vi "Begin.vi"(8 "error in":errorcluster) -> (0 "error out":errorcluster)   [LabVIEW 2015]
doc: "Called before other user functions, this VI is expected to open initial I/O refnums, load in file data, and do all program initialization. Notice that the <B>error out</B> terminal is simply used for data flow. Wiring it to other structures or subVIs ensures that this VI runs first."
uses:
  <vilib>/Rock Robotics/WPI/DriverStation/WPI_DriverStationRobotMode2.ctl
  <vilib>/Rock Robotics/WPI/Joystick/WPI_JoystickDeviceEnum.ctl
  <vilib>/Rock Robotics/WPI/Solenoid/WPI_SolenoidChannel.ctl
  <vilib>/Rock Robotics/WPI/CAN/TalonSRX/WPI_CANTalonSRX_APIControlMode.ctl
  <vilib>/Rock Robotics/WPI/CAN/TalonSRX/WPI_CANTalonSRX_BrakeOverride.ctl
  <vilib>/Rock Robotics/SystemInterfaces/AI/FPGA_AIChannel.ctl
  <vilib>/Rock Robotics/SystemInterfaces/DIO/FPGA_DIOChannel.ctl
  <vilib>/Rock Robotics/SystemInterfaces/DIO/FPGA_DIOPWMChannel.ctl
  <vilib>/Rock Robotics/WPI/CAN/TalonSRX/WPI_CANTalonSRX_APIFeedbackSelect.ctl
  <vilib>/Rock Robotics/SystemInterfaces/spilib/spi_bus.ctl
  navX-MXP Library/COMMON/TypeDefs/Value TypeDefs/navX Interface Protocol.ctl
  navX-MXP Library/COMMON/TypeDefs/Value TypeDefs/navX Update Rate.ctl
  Robot Global Data.vi
  <vilib>/Rock Robotics/WPI/Utilities/WPI_GetSetVariantRefNum.vi
  <vilib>/Rock Robotics/WPI/Solenoid/WPI_SolenoidOpenSingle.vi
  <vilib>/Rock Robotics/WPI/MotorControl/WPI_MotorControlOpenCANTalonSRX.vi
  <vilib>/Rock Robotics/WPI/Ultrasonic/WPI_SonarSRF04DigitalOpen.vi
  <vilib>/Rock Robotics/WPI/Ultrasonic/WPI_SonarSRF04DigitalRefNum Registry Set.vi
  <vilib>/Rock Robotics/WPI/MotorControl/WPI_MotorControlOpen VictorSP.vi
  <vilib>/Rock Robotics/WPI/Counter/WPI_CounterDigitalInputToDigitalSource.vi
  <vilib>/Rock Robotics/WPI/Camera/WPI_CameraWhite Balance Values.ctl
  <vilib>/Rock Robotics/WPI/Camera/WPI_CameraExposure Values.ctl
  navX-MXP Library/navX-MXP IMU.lvlib
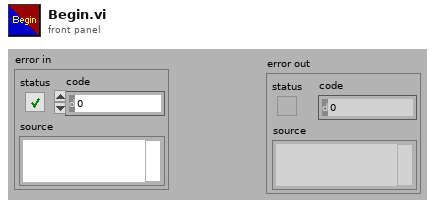
[diagram p1: front panel]
types:
  T1 = typedef "WPI_CANTalonSRX_APIFeedbackSelect.ctl" = enum16{"Digital Quadrature Encoder", "Analog Potentiometer", "Analog Encoder", "Count on Quad-A (Rising-Edge)", "Count on Quad-A (Falling-Edge)", "CTR Magnetic Enc (Absolute)", "CTR Magnetic Enc (Relative)", "Pulse Width"}
  T2 = typedef "FPGA_DIOPWMChannel.ctl" = enum8{"PWM 0", "PWM 1", "PWM 2", "PWM 3", "PWM 4", "PWM 5", "PWM 6", "PWM 7", "PWM 8", "PWM 9", "PWM MXP 0", "PWM MXP 1", "PWM MXP 2", "PWM MXP 3", "PWM MXP 4", "PWM MXP 5", "PWM MXP 6", "PWM MXP 7", "PWM MXP 8", "PWM MXP 9", "Invalid"}
  T3 = typedef "FPGA_DIOChannel.ctl" = enum8{"DIO 0", "DIO 1", "DIO 2", "DIO 3", "DIO 4", "DIO 5", "DIO 6", "DIO 7", "DIO 8", "DIO 9", "DIO MXP 0", "DIO MXP 1", "DIO MXP 2", "DIO MXP 3", "DIO MXP 4", "DIO MXP 5", "DIO MXP 6", "DIO MXP 7", "DIO MXP 8", "DIO MXP 9", "DIO MXP 10", "DIO MXP 11", "DIO MXP 12", "DIO MXP 13", "DIO MXP 14", "DIO MXP 15", "Invalid"}
  T4 = typedef "WPI_CANTalonSRX_BrakeOverride.ctl" = enum8{"No Override", "Override to Coast", "Override to Brake"}
  T5 = typedef "WPI_SolenoidChannel.ctl" = enum8{"Solenoid 0", "Solenoid 1", "Solenoid 2", "Solenoid 3", "Solenoid 4", "Solenoid 5", "Solenoid 6", "Solenoid 7", "Invalid"}
  T6 = typedef "WPI_CANTalonSRX_APIControlMode.ctl" = enum8{"Percent VBus", "Speed", "Position", "Slave", "Unchanged / Invalid", "Voltage Compensation", "Current", "Motion Profile"}
  T7 = typedef "FPGA_AIChannel.ctl" = enum8{"AI 0", "AI 1", "AI 2", "AI 3", "AI MXP 0", "AI MXP 1", "AI MXP 2", "AI MXP 3", "Invalid"}
  T8 = typedef "WPI_JoystickDeviceEnum.ctl" = enum16{"USB 0", "USB 1", "USB 2", "USB 3", "USB 4", "USB 5"}
  T9 = typedef "WPI_DriverStationRobotMode2.ctl" = enum16{"Autonomous Disabled", "Autonomous Enabled", "Teleop Disabled", "Teleop Enabled", "Disconnected", "Finish", "Test Disabled", "Test Enabled", "Emergency Stopped"}
  T10 = typedef "navX-MXP IMU.lvlib/navX Update Rate.ctl" = u8
  T11 = typedef "navX-MXP IMU.lvlib/navX Interface Protocol.ctl" = enum16{"SPI", "I2C"}
  T12 = typedef "spi_bus.ctl" = enum16{"SPI On-Board, CS0", "SPI On-Board, CS1", "SPI On-Board, CS2", "SPI On-Board, CS3", "SPI MXP", "Invalid"}
  T13 = typedef "navX-MXP IMU.lvlib/navX Device TypeDef.ctl" = cluster{"navX Interface Protocol":T11, "navX Interface Protocol TypeDefs":cluster{"SPIDevRef":T14, "I2CDevRef":T15}, "navX System Information":cluster{"Board Information":T17, "Status":T18, "Offsets":T22}, "navX Common Information":cluster{"Update Rate (4Hz-60Hz)":T10, "refnum name":string, "error":errorcluster}}
  T14 = typedef "WPI_SPIDevRef.ctl" = cluster{"DevStatus":errorcluster, "Handle":i32, "SPI Bus":T12}
  T15 = typedef "WPI_I2CDevRef.ctl" = cluster{"DevStatus":errorcluster, "Device Address":u8, "Handle":i32, "I2C Bus":T16}
  T16 = typedef "i2c_bus.ctl" = enum16{"I2C On-Board", "I2C MXP", "Invalid"}
  T17 = typedef "navX-MXP IMU.lvlib/navX Board Information.ctl" = cluster{"WhoAmI (50 | 0x32)":u8, "Board Revision":u8, "Firmware Major Version":u8, "Firmware Minor Version":u8}
  T18 = typedef "navX-MXP IMU.lvlib/navX Status Data.ctl" = cluster{"Update Rate Hz":u8, "Accelerometer Full-Scale Range":u8, "Gyro Full-Scale Range":u16, "NAVX_OP_STATUS":T19, "NAVX_CAL_STATUS":T20, "NAVX_SELFTEST_STATUS":u8, "NAVX_SENSOR_STATUS":T21}
  T19 = typedef "navX-MXP IMU.lvlib/navX NAVX_OP_STATUS.ctl" = u8
  T20 = typedef "navX-MXP IMU.lvlib/navX NAVX_CAL_STATUS.ctl" = u8
  T21 = typedef "navX-MXP IMU.lvlib/navX NAVX_SENSOR_STATUS.ctl" = cluster{"MOVING":bool, "YAW_STABLE":bool, "MAG_DISTURBANCE":bool, "ALTITUDE_VALID":bool, "SEALEVEL_PRESS_SET":bool, "FUSED_HEADING_VALID":bool}
  T22 = typedef "navX-MXP IMU.lvlib/navX Offsets Data.ctl" = cluster{"Yaw":dbl, "Quat W":dbl, "Quat X":dbl, "Quat Y":dbl, "Quat Z":dbl}
  T23 = typedef "WPI_CameraExposure Values.ctl" = enum16{"Auto", "Flicker-free 50 Hz", "Flicker-free 60 Hz", "Hold current", "Custom"}
  T24 = typedef "WPI_CameraWhite Balance Values.ctl" = enum16{"Auto", "Fixed indoor", "Fixed outdoor 1", "Fixed outdoor 2", "Fixed fluorescent 1", "Fixed fluorescent 2", "Hold current", "Custom"}
  T25 = typedef "WPI_CameraDevRef.ctl" = cluster{"Camera Address":string, "CameraStatus":errorcluster}
  T26 = typedef "WPI_DigitalInputDevRef.ctl" = cluster{"DevStatus":errorcluster, "DIO Channel":T3}
  T27 = typedef "FPGA_CounterEncoderSourceConvertionLVSourceType.ctl" = cluster{"DevStatus":errorcluster, "AnalogTriggerMode?":bool, "DigitalMode":cluster{"DIO Channel":T28}, "AnalogTriggerMode":cluster{"AnalogTriggerIndex":T29, "OutputType":T30}}
  T28 = typedef "FPGA_DIODigitalSourceChannel.ctl" = enum8{"DIO 0", "DIO 1", "DIO 2", "DIO 3", "DIO 4", "DIO 5", "DIO 6", "DIO 7", "DIO 8", "DIO 9", "DIO MXP 0", "DIO MXP 1", "DIO MXP 2", "DIO MXP 3", "DIO MXP 4", "DIO MXP 5", "DIO MXP 6", "DIO MXP 7", "DIO MXP 8", "DIO MXP 9", "DIO MXP 10", "DIO MXP 11", "DIO MXP 12", "DIO MXP 13", "DIO MXP 14", "DIO MXP 15", "Disabled"}
  T29 = typedef "FPGA_AnalogTriggerIndex.ctl" = enum8{"Trig 0", "Trig 1", "Trig 2", "Trig 3", "Trig 4", "Trig 5", "Trig 6", "Trig 7", "Invalid"}
  T30 = typedef "FPGA_AnalogTriggerOutType.ctl" = enum16{"InWindow", "TriggerState", "Rising", "Falling"}
  T31 = typedef "WPI_EncoderDevRef.ctl" = cluster{"DevStatus":errorcluster, "EncoderIndex":T32, "CounterIndex":T33, "DistancePerCount":dbl, "Decoding Type":T34}
  T32 = typedef "FPGA_EncoderIdx.ctl" = enum8{"Enc 0", "Enc 1", "Enc 2", "Enc 3", "Enc 4", "Enc 5", "Enc 6", "Enc 7", "Invalid"}
  T33 = typedef "FPGA_CounterCtrSystemIndex.ctl" = enum8{"Ctr 0", "Ctr 1", "Ctr 2", "Ctr 3", "Ctr 4", "Ctr 5", "Ctr 6", "Ctr 7", "Invalid"}
  T34 = typedef "WPI_EncoderType.ctl" = enum16{"1x", "2x", "4x"}
  T35 = typedef "WPI_UltrasonicDeviceRef.ctl" = cluster{"DevStatus":errorcluster, "Ping Channel":T3, "Echo Channel":T3, "CntIndex":T33}
  T36 = typedef "WPI_SolenoidDevRef.ctl" = cluster{"DevStatus":errorcluster, "Pneumatics Control Module":u8, "Forward Solenoid Channel":T5, "Reverse Solenoid Channel":T5}
  T37 = typedef "WPI_CompressorDevRef.ctl" = cluster{"DevStatus":errorcluster, "Pneumatics Control Module":u8}
  T38 = typedef "WPI_JoystickDevRef.ctl" = cluster{"Device":T8}
  T39 = typedef "WPI_MotorControlDeviceRef.ctl" = cluster{"DeviceStatus":errorcluster, "Type":T40, "PWM":cluster{"PWM Channel":T2, "DeadBand":T41}, "CAN":cluster{"Device Number":u8, "Control Mode":T42, "Semaphore":T43, "Max Vout":dbl, "TalonSRX Control Mode":T6}, "Invert":bool}
  T40 = typedef "WPI_MotorControlType.ctl" = enum16{"PWM", "CAN", "CANTalonSRX"}
  T41 = typedef "WPI_PWMDeadband.ctl" = cluster{"Name":string, "maxPositivePwm":i32, "minPositivePwm":i32, "centerPwm":i32, "maxNegativePwm":i32, "minNegativePwm":i32, "angularRange":u16}
  T42 = typedef "WPI_CANJaguar_ControlMode.ctl" = enum8{"Percent VBus", "Current", "Speed", "Position", "Voltage"}
  T43 = typedef "Semaphore RefNum" = refnum<k1>
  T44 = typedef "WPI_ServoDeviceRef.ctl" = cluster{"DeviceStatus":errorcluster, "PWM Channel":T2, "DeadBand":T41}
  T45 = typedef "WPI_PotentiometerDevRef.ctl" = cluster{"DevStatus":errorcluster, "Analog Channel":T7, "Invert Output":bool}
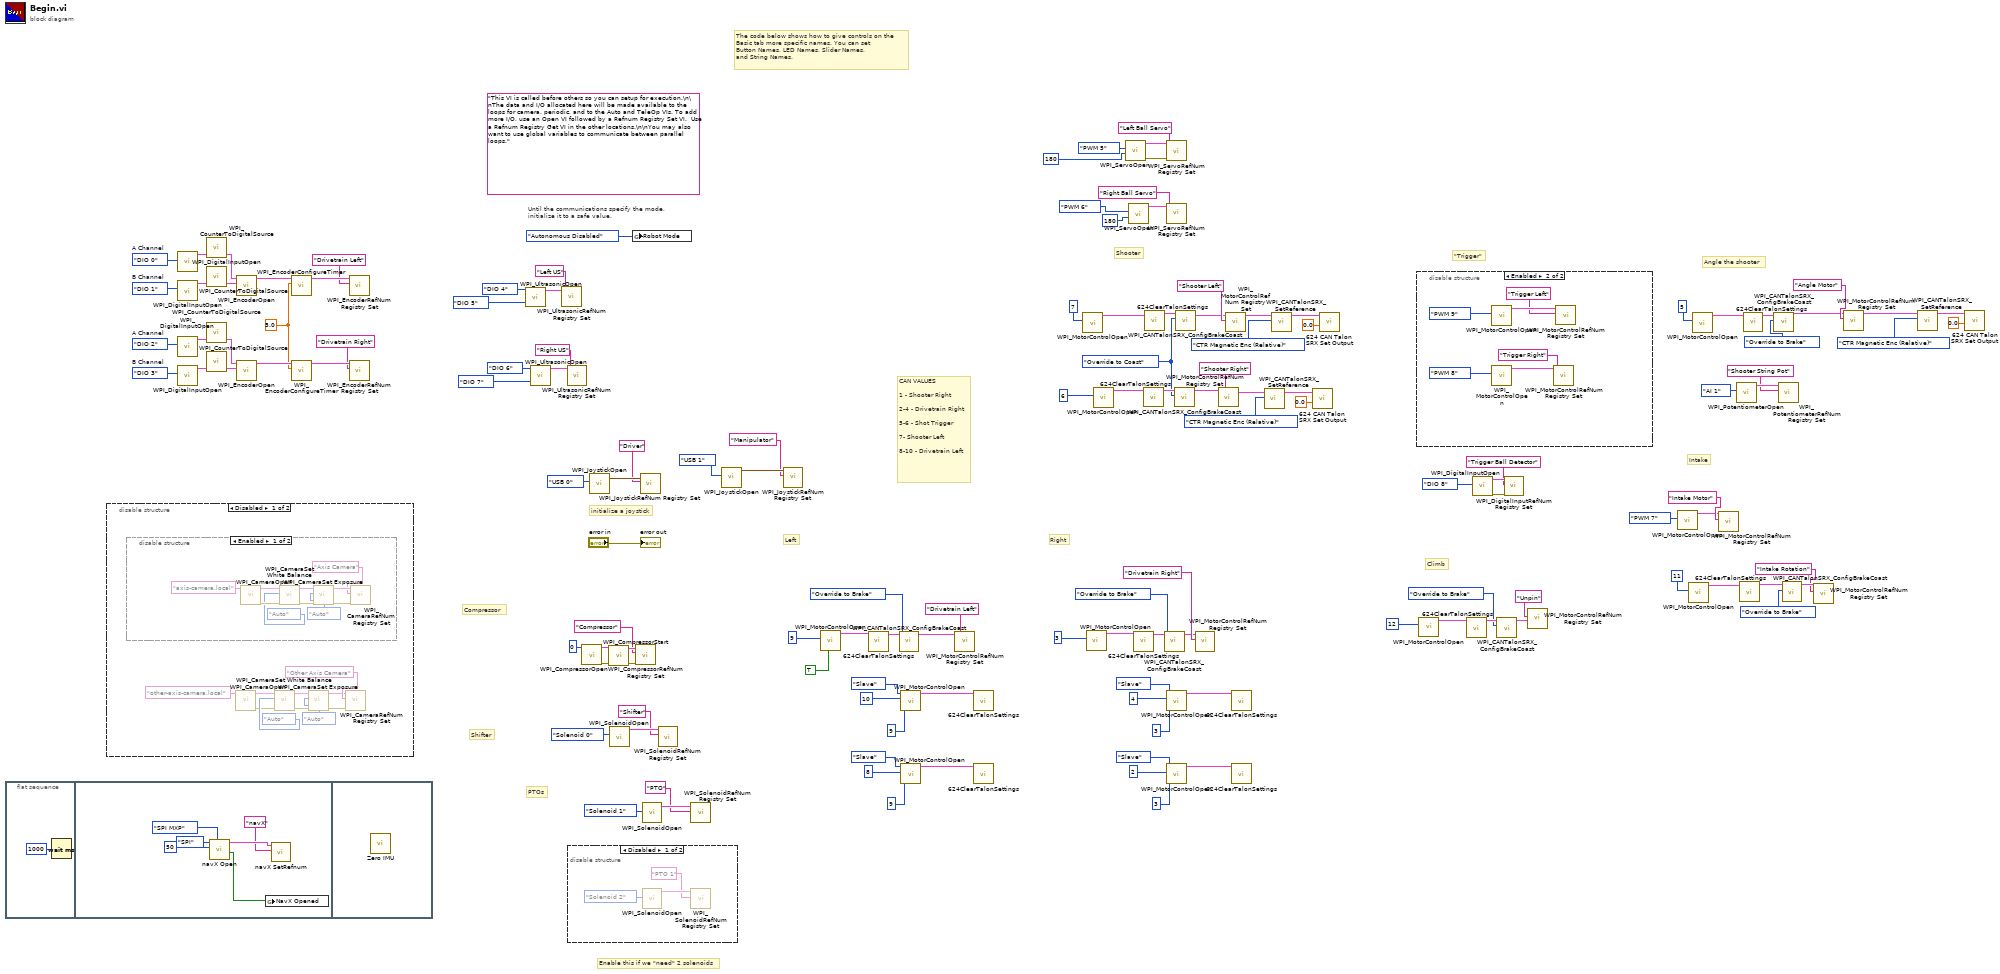
[diagram p0: block diagram]
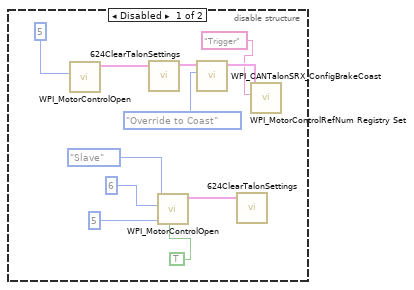
[diagram p2: hidden frame]
diagram:
  w26 = FPGA_DIOChannel."DIO 3"  # B Channel
  w29 = FPGA_DIOChannel."DIO 0"  # A Channel
  w32 = FPGA_DIOChannel."DIO 1"  # B Channel
  w37 = 5.0 ("Minimum Rate")
  w40 = FPGA_DIOChannel."DIO 2"  # A Channel
  w64 = WPI_CANTalonSRX_BrakeOverride."Override to Coast" ("Brake / Coast Mode")
  (unwired) "This VI is called before others so you can setup for execution.\n\nThe data and I/O allocated here will be made available to the loops for camera, periodic, and to the Auto and TeleOp VIs. To add more I/O, use an Open VI followed by a Refnum Registry Set VI.  Use a Refnum Registry Get VI in the other locations.\n\nYou may also want to use global variables to communicate between parallel loops."
  # "Climb"
  # "Enable this if we \"need\" 2 solenoids"
  # "CAN VALUES\n\n1 - Shooter Right\n\n2-4 - Drivetrain Right\n\n5-6 - Shot Trigger\n\n7- Shooter Left\n\n8-10 - Drivetrain Left"
  # "Angle the shooter"
  # "PTOs"
  # "Intake"
  # "\"Trigger\""
  # "Shooter"
  # "Left"
  # "Right"
  # "Shifter"
  # "Compressor"
  # "The code below shows how to give controls on the\nBasic tab more specific names. You can set\nButton Names, LED Names, Slider Names,\nand String Names."
  # "initialize a joystick"
  # "Until the communications specify the mode,\ninitialize it to a safe value."
  n1 = flat-sequence {
    frame #0 {
      n2 = Wait (ms)(milliseconds to wait=u32 1000) -> ()  [unwired: 1 out]
    }
    frame #1 {
      n3 = call "navX Open.vi"("SPI Bus"=spi_bus."SPI MXP", "Update Rate (4Hz-60Hz)"=T10 50, "navX Interface Protocol"=navX_Interface_Protocol."SPI") -> ("Opened?"=w138:bool, "navX Device TypeDef"=w140:T13)  [unwired: 6 in, 1 out]
      n4 = global write "Robot Global Data.vi" "NavX Opened"(w138) -> ()
      n5 = call "navX SetRefnum.vi"("refnum name"="navX", "navX Device TypeDef"=w140) -> ()  [unwired: 8 in, 2 out]
    }
    frame #2 {
      n6 = call "Zero IMU.vi"() -> ()  [unwired: 12 in]
    }
  }
  n7 = disable-structure shown="Disabled" {
    frame Disabled {
      n8 = disable-structure shown="Enabled" {
        frame Enabled {
          n9 = call <vilib>:"WPI_CameraOpen.vi"("Camera Address"="axis-camera.local") -> ("error out"=w159:errorcluster, "CameraDevRef"=w158:T25)  [unwired: 9 in]
          n10 = call <vilib>:"WPI_CameraSet White Balance.vi"("error in (no error)"=w159, "White Balance"=WPI_CameraWhite_Balance_Values."Auto", "CameraDevRef"=w158) -> ("error out"=w161:errorcluster, "CameraDevRef Out"=w160:T25)  [unwired: 7 in]
          n11 = call <vilib>:"WPI_CameraSet Exposure.vi"("error in (no error)"=w161, "Exposure"=WPI_CameraExposure_Values."Auto", "CameraDevRef"=w160) -> ("error out"=w163:errorcluster, "CameraDevRef Out"=w162:T25)  [unwired: 7 in]
          n12 = call <vilib>:"WPI_CameraRefNum Registry Set.vi"("error in (no error)"=w163, "refnum name"="Axis Camera", "CameraDevRef"=w162) -> ()  [unwired: 7 in, 2 out]
        }
        frame Disabled {
        }
      }
      n13 = call <vilib>:"WPI_CameraOpen.vi"("Camera Address"="other-axis-camera.local") -> ("error out"=w148:errorcluster, "CameraDevRef"=w149:T25)  [unwired: 9 in]
      n14 = call <vilib>:"WPI_CameraSet White Balance.vi"("error in (no error)"=w148, "White Balance"=WPI_CameraWhite_Balance_Values."Auto", "CameraDevRef"=w149) -> ("error out"=w146:errorcluster, "CameraDevRef Out"=w147:T25)  [unwired: 7 in]
      n15 = call <vilib>:"WPI_CameraSet Exposure.vi"("error in (no error)"=w146, "Exposure"=WPI_CameraExposure_Values."Auto", "CameraDevRef"=w147) -> ("error out"=w144:errorcluster, "CameraDevRef Out"=w145:T25)  [unwired: 7 in]
      n16 = call <vilib>:"WPI_CameraRefNum Registry Set.vi"("error in (no error)"=w144, "refnum name"="Other Axis Camera", "CameraDevRef"=w145) -> ()  [unwired: 7 in, 2 out]
    }
    frame Enabled {
    }
  }
  n17 = call <vilib>:"WPI_DigitalInputOpen.vi"("DIO Channel"=w29) -> ("DigitalInputDevRef"=w30:T26)  [unwired: 1 in, 9 out]
  n18 = call <vilib>:"WPI_DigitalInputOpen.vi"("DIO Channel"=w32) -> ("DigitalInputDevRef"=w33:T26)  [unwired: 1 in, 9 out]
  n19 = call <vilib>:"WPI_DigitalInputOpen.vi"("DIO Channel"=w40) -> ("DigitalInputDevRef"=w41:T26)  [unwired: 1 in, 9 out]
  n20 = call <vilib>:"WPI_DigitalInputOpen.vi"("DIO Channel"=w26) -> ("DigitalInputDevRef"=w38:T26)  [unwired: 1 in, 9 out]
  n21 = call-poly <vilib>:"WPI_CounterToDigitalSource.vi"("DigitalInputDevRef"=w30) -> ("Digital Source"=w31:T27)  [unwired: 6 out]
  n22 = call-poly <vilib>:"WPI_CounterToDigitalSource.vi"("DigitalInputDevRef"=w33) -> ("Digital Source"=w34:T27)  [unwired: 6 out]
  n23 = call-poly <vilib>:"WPI_CounterToDigitalSource.vi"("DigitalInputDevRef"=w41) -> ("Digital Source"=w42:T27)  [unwired: 6 out]
  n24 = call-poly <vilib>:"WPI_CounterToDigitalSource.vi"("DigitalInputDevRef"=w38) -> ("Digital Source"=w39:T27)  [unwired: 6 out]
  n25 = call <vilib>:"WPI_EncoderOpen.vi"("BSource"=w34, "ASource"=w31) -> ("EncoderDevRef"=w35:T31)  [unwired: 6 in, 3 out]
  n26 = call <vilib>:"WPI_EncoderOpen.vi"("BSource"=w39, "ASource"=w42) -> ("EncoderDevRef"=w43:T31)  [unwired: 6 in, 3 out]
  n27 = call <vilib>:"WPI_EncoderConfigureTimer.vi"("Minimum Rate"=w37, "EncoderDevRef"=w35) -> ("EncoderDevRef"=w36:T31)  [unwired: 8 in, 1 out]
  n28 = call <vilib>:"WPI_EncoderConfigureTimer.vi"("Minimum Rate"=w37, "EncoderDevRef"=w43) -> ("EncoderDevRef"=w44:T31)  [unwired: 8 in, 1 out]
  n29 = call <vilib>:"WPI_EncoderRefNum Registry Set.vi"("refnum name"="Drivetrain Left", "EncoderDevRef"=w36) -> ()  [unwired: 8 in, 2 out]
  n30 = call <vilib>:"WPI_EncoderRefNum Registry Set.vi"("refnum name"="Drivetrain Right", "EncoderDevRef"=w44) -> ()  [unwired: 8 in, 2 out]
  n31 = call-poly <vilib>:"WPI_UltrasonicOpen.vi"("Echo DIO Channel"=FPGA_DIOChannel."DIO 5", "Ping DIO Channel"=FPGA_DIOChannel."DIO 4") -> ("SonarSRF04DevRef"=w58:T35)  [unwired: 8 in, 1 out]
  n32 = call-poly <vilib>:"WPI_UltrasonicOpen.vi"("Echo DIO Channel"=FPGA_DIOChannel."DIO 7", "Ping DIO Channel"=FPGA_DIOChannel."DIO 6") -> ("SonarSRF04DevRef"=w51:T35)  [unwired: 8 in, 1 out]
  n33 = call-poly <vilib>:"WPI_UltrasonicRefNum Registry Set.vi"("refnum name"="Left US", "SonarSRF04DevRef"=w58) -> ()  [unwired: 8 in, 2 out]
  n34 = call-poly <vilib>:"WPI_UltrasonicRefNum Registry Set.vi"("refnum name"="Right US", "SonarSRF04DevRef"=w51) -> ()  [unwired: 8 in, 2 out]
  n35 = disable-structure shown="Disabled" {
    frame Disabled {
      n36 = call-poly <vilib>:"WPI_SolenoidOpen.vi"("Solenoid Channel"=WPI_SolenoidChannel."Solenoid 2") -> ("SolenoidDevRef"=w166:T36)  [unwired: 9 in, 1 out]
      n37 = call <vilib>:"WPI_SolenoidRefNum Registry Set.vi"("refnum name"="PTO 1", "SolenoidDevRef"=w166) -> ()  [unwired: 8 in, 2 out]
    }
    frame Enabled {
    }
  }
  n38 = call <vilib>:"WPI_CompressorOpen.vi"("Pneumatics Control Module (0)"=0) -> ("CompressorDevRef"=w131:T37, "error out"=w128:errorcluster)  [unwired: 13 in]
  n39 = call <vilib>:"WPI_JoystickOpen.vi"("JoystickDevice"=WPI_JoystickDeviceEnum."USB 0") -> ("JoystickDevRef"=w135:T38)  [unwired: 10 in]
  n40 = call <vilib>:"WPI_CompressorStart.vi"("error in (no error)"=w128, "CompressorDevRef"=w131) -> ("error out"=w127:errorcluster, "CompressorDevRef"=w130:T37)  [unwired: 8 in]
  n41 = call-poly <vilib>:"WPI_SolenoidOpen.vi"("Solenoid Channel"=WPI_SolenoidChannel."Solenoid 0") -> ("SolenoidDevRef"=w125:T36)  [unwired: 9 in, 1 out]
  n42 = global write "Robot Global Data.vi" "Robot Mode"(WPI_DriverStationRobotMode2."Autonomous Disabled" ("Robot Mode")) -> ()
  n43 = call <vilib>:"WPI_CompressorRefNum Registry Set.vi"("error in (no error)"=w127, "refnum name"="Compressor", "CompressorDevRef"=w130) -> ()  [unwired: 7 in, 2 out]
  n44 = call <vilib>:"WPI_JoystickRefNum Registry Set.vi"("refnum name"="Driver", "JoystickDevRef"=w135) -> ()  [unwired: 8 in, 2 out]
  n45 = call-poly <vilib>:"WPI_SolenoidOpen.vi"("Solenoid Channel"=WPI_SolenoidChannel."Solenoid 1") -> ("SolenoidDevRef"=w70:T36)  [unwired: 9 in, 1 out]
  n46 = call <vilib>:"WPI_SolenoidRefNum Registry Set.vi"("refnum name"="Shifter", "SolenoidDevRef"=w125) -> ()  [unwired: 8 in, 2 out]
  n47 = call <vilib>:"WPI_SolenoidRefNum Registry Set.vi"("refnum name"="PTO", "SolenoidDevRef"=w70) -> ()  [unwired: 8 in, 2 out]
  n48 = call <vilib>:"WPI_JoystickOpen.vi"("JoystickDevice"=WPI_JoystickDeviceEnum."USB 1") -> ("JoystickDevRef"=w100:T38)  [unwired: 10 in]
  n49 = call <vilib>:"WPI_JoystickRefNum Registry Set.vi"("refnum name"="Manipulator", "JoystickDevRef"=w100) -> ()  [unwired: 8 in, 2 out]
  n50 = call-poly <vilib>:"WPI_MotorControlOpen.vi"("Invert"=TRUE, "Device Number"=9) -> ("MotorControlDeviceRef"=w104:T39)  [unwired: 8 in, 1 out]
  n51 = call "624ClearTalonSettings.vi"("MotorControlDeviceRef 2"=w104) -> ("MotorControlDeviceRef"=w105:T39)  [unwired: 10 in]
  n52 = call <vilib>:"WPI_CANTalonSRX_ConfigBrakeCoast.vi"("Brake / Coast Mode"=WPI_CANTalonSRX_BrakeOverride."Override to Brake", "CAN Talon SRX Ref"=w105) -> ("CAN Talon SRX Ref"=w16:T39)  [unwired: 8 in, 1 out]
  n53 = call-poly <vilib>:"WPI_MotorControlOpen.vi"("Master Device Number"=u8 9, "Device Number"=u8 10, "Control Mode"=WPI_CANTalonSRX_APIControlMode."Slave") -> ("MotorControlDeviceRef"=w109:T39)  [unwired: 7 in, 1 out]
  n54 = call-poly <vilib>:"WPI_MotorControlOpen.vi"("Master Device Number"=u8 9, "Device Number"=u8 8, "Control Mode"=WPI_CANTalonSRX_APIControlMode."Slave") -> ("MotorControlDeviceRef"=w110:T39)  [unwired: 7 in, 1 out]
  n55 = call <vilib>:"WPI_MotorControlRefNum Registry Set.vi"("refnum name"="Drivetrain Left", "MotorControlDevRef"=w16) -> ()  [unwired: 8 in, 2 out]
  n56 = call "624ClearTalonSettings.vi"("MotorControlDeviceRef 2"=w109) -> ()  [unwired: 10 in, 1 out]
  n57 = call "624ClearTalonSettings.vi"("MotorControlDeviceRef 2"=w110) -> ()  [unwired: 10 in, 1 out]
  n58 = call-poly <vilib>:"WPI_MotorControlOpen.vi"("Device Number"=u8 7) -> ("MotorControlDeviceRef"=w62:T39)  [unwired: 9 in, 1 out]
  n59 = call-poly <vilib>:"WPI_MotorControlOpen.vi"("Device Number"=3) -> ("MotorControlDeviceRef"=w120:T39)  [unwired: 9 in, 1 out]
  n60 = call-poly <vilib>:"WPI_MotorControlOpen.vi"("Device Number"=u8 6) -> ("MotorControlDeviceRef"=w66:T39)  [unwired: 9 in, 1 out]
  n61 = call <vilib>:"WPI_ServoOpen.vi"("Angular Range"=u16 180, "PWM Channel"=FPGA_DIOPWMChannel."PWM 5") -> ("error out"=w23:errorcluster, "ServoDeviceRef"=w22:T44)  [unwired: 8 in]
  n62 = call <vilib>:"WPI_ServoOpen.vi"("Angular Range"=u16 180, "PWM Channel"=FPGA_DIOPWMChannel."PWM 6") -> ("ServoDeviceRef"=w21:T44)  [unwired: 8 in, 1 out]
  n63 = call "624ClearTalonSettings.vi"("MotorControlDeviceRef 2"=w120) -> ("MotorControlDeviceRef"=w119:T39)  [unwired: 10 in]
  n64 = call "624ClearTalonSettings.vi"("MotorControlDeviceRef 2"=w66) -> ("MotorControlDeviceRef"=w67:T39)  [unwired: 10 in]
  n65 = call "624ClearTalonSettings.vi"("MotorControlDeviceRef 2"=w62) -> ("MotorControlDeviceRef"=w63:T39)  [unwired: 10 in]
  n66 = call <vilib>:"WPI_CANTalonSRX_ConfigBrakeCoast.vi"("Brake / Coast Mode"=WPI_CANTalonSRX_BrakeOverride."Override to Brake", "CAN Talon SRX Ref"=w119) -> ("CAN Talon SRX Ref"=w118:T39)  [unwired: 8 in, 1 out]
  n67 = call <vilib>:"WPI_ServoRefNum Registry Set.vi"("error in (no error)"=w23, "refnum name"="Left Ball Servo", "ServoDeviceRef"=w22) -> ()  [unwired: 7 in, 2 out]
  n68 = call-poly <vilib>:"WPI_MotorControlOpen.vi"("Master Device Number"=u8 3, "Device Number"=u8 4, "Control Mode"=WPI_CANTalonSRX_APIControlMode."Slave") -> ("MotorControlDeviceRef"=w71:T39)  [unwired: 7 in, 1 out]
  n69 = call-poly <vilib>:"WPI_MotorControlOpen.vi"("Master Device Number"=u8 3, "Device Number"=u8 2, "Control Mode"=WPI_CANTalonSRX_APIControlMode."Slave") -> ("MotorControlDeviceRef"=w117:T39)  [unwired: 7 in, 1 out]
  n70 = call <vilib>:"WPI_ServoRefNum Registry Set.vi"("refnum name"="Right Ball Servo", "ServoDeviceRef"=w21) -> ()  [unwired: 8 in, 2 out]
  n71 = call <vilib>:"WPI_CANTalonSRX_ConfigBrakeCoast.vi"("Brake / Coast Mode"=w64, "CAN Talon SRX Ref"=w67) -> ("CAN Talon SRX Ref"=w12:T39)  [unwired: 8 in, 1 out]
  n72 = call <vilib>:"WPI_CANTalonSRX_ConfigBrakeCoast.vi"("Brake / Coast Mode"=w64, "CAN Talon SRX Ref"=w63) -> ("CAN Talon SRX Ref"=w13:T39)  [unwired: 8 in, 1 out]
  n73 = call <vilib>:"WPI_MotorControlRefNum Registry Set.vi"("refnum name"="Drivetrain Right", "MotorControlDevRef"=w118) -> ()  [unwired: 8 in, 2 out]
  n74 = call <vilib>:"WPI_MotorControlRefNum Registry Set.vi"("refnum name"="Shooter Right", "MotorControlDevRef"=w12) -> ("MotorControlDevRef"=w15:T39)  [unwired: 8 in, 1 out]
  n75 = call <vilib>:"WPI_MotorControlRefNum Registry Set.vi"("refnum name"="Shooter Left", "MotorControlDevRef"=w13) -> ("MotorControlDevRef"=w7:T39)  [unwired: 8 in, 1 out]
  n76 = call "624ClearTalonSettings.vi"("MotorControlDeviceRef 2"=w71) -> ()  [unwired: 10 in, 1 out]
  n77 = call "624ClearTalonSettings.vi"("MotorControlDeviceRef 2"=w117) -> ()  [unwired: 10 in, 1 out]
  n78 = call <vilib>:"WPI_CANTalonSRX_SetReference.vi"("Feedback Reference"=WPI_CANTalonSRX_APIFeedbackSelect."CTR Magnetic Enc (Relative)", "CAN Talon SRX Ref"=w15) -> ("CAN Talon SRX Ref"=w11:T39)  [unwired: 8 in, 1 out]
  n79 = call <vilib>:"WPI_CANTalonSRX_SetReference.vi"("Feedback Reference"=WPI_CANTalonSRX_APIFeedbackSelect."CTR Magnetic Enc (Relative)", "CAN Talon SRX Ref"=w7) -> ("CAN Talon SRX Ref"=w8:T39)  [unwired: 8 in, 1 out]
  n80 = call "624 CAN Talon SRX Set Output.vi"("Output"=0.0, "MotorControlDevRef"=w11) -> ()  [unwired: 9 in, 1 out]
  n81 = call "624 CAN Talon SRX Set Output.vi"("Output"=0.0, "MotorControlDevRef"=w8) -> ()  [unwired: 9 in, 1 out]
  n82 = disable-structure shown="Enabled" {
    frame Disabled {
      n83 = call-poly <vilib>:"WPI_MotorControlOpen.vi"("Device Number"=u8 5) -> ("MotorControlDeviceRef"=w176:T39)  [unwired: 9 in, 1 out]
      n84 = call "624ClearTalonSettings.vi"("MotorControlDeviceRef 2"=w176) -> ("MotorControlDeviceRef"=w175:T39)  [unwired: 10 in]
      n85 = call-poly <vilib>:"WPI_MotorControlOpen.vi"("Invert"=TRUE, "Master Device Number"=u8 5, "Device Number"=u8 6, "Control Mode"=WPI_CANTalonSRX_APIControlMode."Slave") -> ("MotorControlDeviceRef"=w171:T39)  [unwired: 6 in, 1 out]
      n86 = call <vilib>:"WPI_CANTalonSRX_ConfigBrakeCoast.vi"("Brake / Coast Mode"=WPI_CANTalonSRX_BrakeOverride."Override to Coast", "CAN Talon SRX Ref"=w175) -> ("CAN Talon SRX Ref"=w174:T39)  [unwired: 8 in, 1 out]
      n87 = call "624ClearTalonSettings.vi"("MotorControlDeviceRef 2"=w171) -> ()  [unwired: 10 in, 1 out]
      n88 = call <vilib>:"WPI_MotorControlRefNum Registry Set.vi"("refnum name"="Trigger", "MotorControlDevRef"=w174) -> ()  [unwired: 8 in, 2 out]
    }
    frame Enabled {
      n89 = call-poly <vilib>:"WPI_MotorControlOpen.vi"("PWM Channel"=FPGA_DIOPWMChannel."PWM 9") -> ("MotorControlDeviceRef"=w181:T39)  [unwired: 9 in, 1 out]
      n90 = call-poly <vilib>:"WPI_MotorControlOpen.vi"("PWM Channel"=FPGA_DIOPWMChannel."PWM 8") -> ("MotorControlDeviceRef"=w180:T39)  [unwired: 9 in, 1 out]
      n91 = call <vilib>:"WPI_MotorControlRefNum Registry Set.vi"("refnum name"="Trigger Right", "MotorControlDevRef"=w180) -> ()  [unwired: 8 in, 2 out]
      n92 = call <vilib>:"WPI_MotorControlRefNum Registry Set.vi"("refnum name"="Trigger Left", "MotorControlDevRef"=w181) -> ()  [unwired: 8 in, 2 out]
    }
  }
  n93 = call-poly <vilib>:"WPI_MotorControlOpen.vi"("Device Number"=12) -> ("MotorControlDeviceRef"=w83:T39)  [unwired: 9 in, 1 out]
  n94 = call "624ClearTalonSettings.vi"("MotorControlDeviceRef 2"=w83) -> ("MotorControlDeviceRef"=w84:T39)  [unwired: 10 in]
  n95 = call <vilib>:"WPI_DigitalInputOpen.vi"("DIO Channel"=FPGA_DIOChannel."DIO 8") -> ("error out"=w49:errorcluster, "DigitalInputDevRef"=w48:T26)  [unwired: 9 in]
  n96 = call <vilib>:"WPI_CANTalonSRX_ConfigBrakeCoast.vi"("Brake / Coast Mode"=WPI_CANTalonSRX_BrakeOverride."Override to Brake", "CAN Talon SRX Ref"=w84) -> ("CAN Talon SRX Ref"=w95:T39)  [unwired: 8 in, 1 out]
  n97 = call <vilib>:"WPI_DigitalInputRefNum Registry Set.vi"("error in (no error)"=w49, "refnum name"="Trigger Ball Detector", "DigitalInputDevRef"=w48) -> ()  [unwired: 7 in, 2 out]
  n98 = call <vilib>:"WPI_MotorControlRefNum Registry Set.vi"("refnum name"="Unpin", "MotorControlDevRef"=w95) -> ()  [unwired: 8 in, 2 out]
  n99 = call-poly <vilib>:"WPI_MotorControlOpen.vi"("PWM Channel"=FPGA_DIOPWMChannel."PWM 7") -> ("MotorControlDeviceRef"=w45:T39)  [unwired: 9 in, 1 out]
  n100 = call-poly <vilib>:"WPI_MotorControlOpen.vi"("Device Number"=u8 11) -> ("MotorControlDeviceRef"=w92:T39)  [unwired: 9 in, 1 out]
  n101 = call-poly <vilib>:"WPI_MotorControlOpen.vi"("Device Number"=u8 5) -> ("MotorControlDeviceRef"=w79:T39)  [unwired: 9 in, 1 out]
  n102 = call <vilib>:"WPI_MotorControlRefNum Registry Set.vi"("refnum name"="Intake Motor", "MotorControlDevRef"=w45) -> ()  [unwired: 8 in, 2 out]
  n103 = call <vilib>:"WPI_PotentiometerOpen.vi"("Analog Channel"=FPGA_AIChannel."AI 1") -> ("PotDevRef"=w88:T45)  [unwired: 9 in, 1 out]
  n104 = call "624ClearTalonSettings.vi"("MotorControlDeviceRef 2"=w92) -> ("MotorControlDeviceRef"=w93:T39)  [unwired: 10 in]
  n105 = call "624ClearTalonSettings.vi"("MotorControlDeviceRef 2"=w79) -> ("MotorControlDeviceRef"=w80:T39)  [unwired: 10 in]
  n106 = call <vilib>:"WPI_CANTalonSRX_ConfigBrakeCoast.vi"("Brake / Coast Mode"=WPI_CANTalonSRX_BrakeOverride."Override to Brake", "CAN Talon SRX Ref"=w80) -> ("CAN Talon SRX Ref"=w2:T39)  [unwired: 8 in, 1 out]
  n107 = call <vilib>:"WPI_PotentiometerRefNum Registry Set.vi"("refnum name"="Shooter String Pot", "PotDevRef"=w88) -> ()  [unwired: 8 in, 2 out]
  n108 = call <vilib>:"WPI_CANTalonSRX_ConfigBrakeCoast.vi"("Brake / Coast Mode"=WPI_CANTalonSRX_BrakeOverride."Override to Brake", "CAN Talon SRX Ref"=w93) -> ("CAN Talon SRX Ref"=w94:T39)  [unwired: 8 in, 1 out]
  n109 = call <vilib>:"WPI_MotorControlRefNum Registry Set.vi"("refnum name"="Intake Rotation", "MotorControlDevRef"=w94) -> ()  [unwired: 8 in, 2 out]
  n110 = call <vilib>:"WPI_MotorControlRefNum Registry Set.vi"("refnum name"="Angle Motor", "MotorControlDevRef"=w2) -> ("MotorControlDevRef"=w1:T39)  [unwired: 8 in, 1 out]
  n111 = call <vilib>:"WPI_CANTalonSRX_SetReference.vi"("Feedback Reference"=WPI_CANTalonSRX_APIFeedbackSelect."CTR Magnetic Enc (Relative)", "CAN Talon SRX Ref"=w1) -> ("CAN Talon SRX Ref"=w4:T39)  [unwired: 8 in, 1 out]
  n112 = call "624 CAN Talon SRX Set Output.vi"("Output"=0.0, "MotorControlDevRef"=w4) -> ()  [unwired: 9 in, 1 out]
  "error out" <- "error in"
